vi "onetoteauto.vi"(8 "error in (no error)":errorcluster) -> (0 "error out":errorcluster)   [LabVIEW 2014]
uses:
  <vilib>/Rock Robotics/WPI/Solenoid/WPI_SolenoidValue.ctl
  <vilib>/Rock Robotics/WPI/RobotDrive/WPI_RobotDriveGetSetRefNum.vi
  <vilib>/Rock Robotics/WPI/RobotDrive/WPI_RobotDriveMecanumDrive_Cartesian.vi
  <vilib>/Rock Robotics/WPI/Solenoid/WPI_SolenoidSetEnum.vi
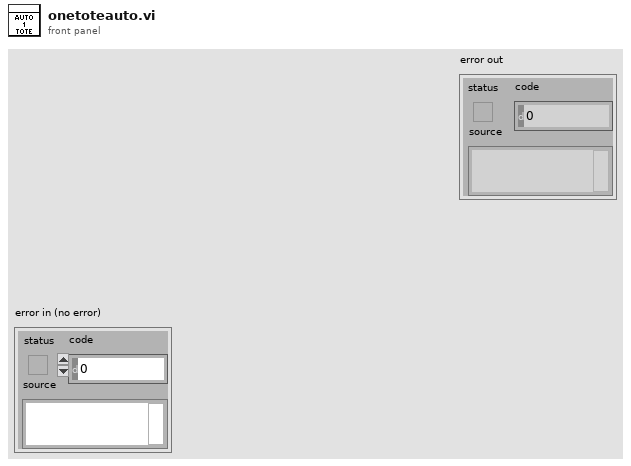
[diagram p1: front panel]
types:
  T1 = typedef "WPI_RobotDriveDevRef.ctl" = cluster{"DevStatus":errorcluster, "Motors[]":T2[], "Square Inputs":bool, "Max Output":dbl}
  T2 = typedef "WPI_MotorControlDeviceRef.ctl" = cluster{"DeviceStatus":errorcluster, "Type":T3, "PWM":cluster{"Controller":T4, "PWM Channel":T5, "DeadBand":T6}, "CAN":cluster{"Device Number":u8, "Control Mode":T7, "Semaphore":T8, "Max Vout":dbl, "TalonSRX Control Mode":T9}, "Invert":bool, "TransformRef":T10, "InvTransformRef":T10}
  T3 = typedef "WPI_MotorControlType.ctl" = enum16{"PWM", "CAN", "CANTalonSRX"}
  T4 = typedef "FPGA_TypedefDigitalModule.ctl" = enum16{"Controller 1"}
  T5 = typedef "FPGA_DIOPWMChannel.ctl" = enum8{"PWM 0", "PWM 1", "PWM 2", "PWM 3", "PWM 4", "PWM 5", "PWM 6", "PWM 7", "PWM 8", "PWM 9", "PWM MXP 0", "PWM MXP 1", "PWM MXP 2", "PWM MXP 3", "PWM MXP 4", "PWM MXP 5", "PWM MXP 6", "PWM MXP 7", "PWM MXP 8", "PWM MXP 9", "Invalid"}
  T6 = typedef "WPI_PWMDeadband.ctl" = cluster{"Name":string, "maxPositivePwm":i32, "minPositivePwm":i32, "centerPwm":i32, "maxNegativePwm":i32, "minNegativePwm":i32, "angularRange":u16}
  T7 = typedef "WPI_CANJaguar_ControlMode.ctl" = enum8{"Percent VBus", "Current", "Speed", "Position", "Voltage"}
  T8 = typedef "Semaphore RefNum" = refnum<k1>
  T9 = typedef "WPI_CANTalonSRX_APIControlMode.ctl" = enum8{"Percent VBus", "Speed", "Position", "Slave", "Unchanged / Invalid"}
  T10 = typedef "WPI_PWMTransform_ConPane.ctl" = refnum<vi>
  T11 = typedef "WPI_SolenoidDevRef.ctl" = cluster{"DevStatus":errorcluster, "Pneumatics Control Module":u8, "Forward Solenoid Channel":T12, "Reverse Solenoid Channel":T12}
  T12 = typedef "WPI_SolenoidChannel.ctl" = enum8{"Solenoid 0", "Solenoid 1", "Solenoid 2", "Solenoid 3", "Solenoid 4", "Solenoid 5", "Solenoid 6", "Solenoid 7", "Invalid"}
  T13 = typedef "WPI_SolenoidValue.ctl" = enum16{"Off", "On", "Forward", "Reverse"}
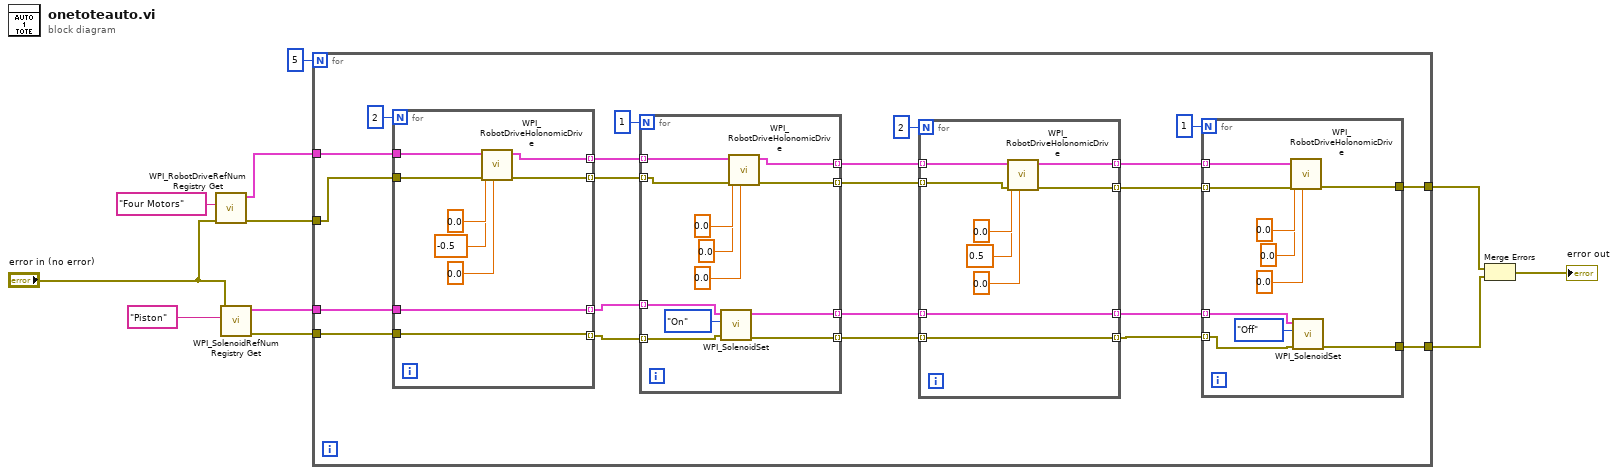
[diagram p0: block diagram]
diagram:
  n1 = call <vilib>:"WPI_RobotDriveRefNum Registry Get.vi"("error in (no error)"="error in (no error)", "refnum name"="Four Motors") -> ("error out"=w8:errorcluster, "RobotDriveDevRef"=w9:T1)  [unwired: 8 in]
  n2 = call <vilib>:"WPI_SolenoidRefNum Registry Get.vi"("error in (no error)"="error in (no error)", "refnum name"="Piston") -> ("error out"=w4:errorcluster, "SolenoidDevRef"=w5:T11)  [unwired: 8 in]
  n3 = for {
    N: 5 -> [_]
    tunnel: w9 -> [w33]
    tunnel: w8 -> [w28]
    tunnel: w5 -> [w24]
    tunnel: w4 -> [w17]
    tunnel: [w13] -> w3
    tunnel: [w12] -> w2
    n4 = for {
      N: 2 -> [_]
      tunnel: w33 -> [w73]
      tunnel: w28 -> [w69]
      tunnel: [w68] -> w27 mode=indexing
      tunnel: [w67] -> w23 mode=indexing
      tunnel: w24 -> [w67]
      tunnel: [w66] -> w20 mode=indexing
      tunnel: [w65] -> w16 mode=indexing
      tunnel: w17 -> [w65]
      n5 = call-poly <vilib>:"WPI_RobotDriveHolonomicDrive.vi"("Rotation"=0.0, "error in (no error)"=w69, "Y"=-0.5, "X"=0.0, "RobotDriveDevRef"=w73) -> ("error out"=w68:errorcluster, "RobotDriveDevRef"=w66:T1)  [unwired: 4 in, 1 out]
    }
    n6 = for {
      N: 1 -> [_]
      tunnel: w27 -> [w61] mode=indexing
      tunnel: [w60] -> w26 mode=indexing
      tunnel: w23 -> [w58] mode=indexing
      tunnel: [w57] -> w21 mode=indexing
      tunnel: w20 -> [w56] mode=indexing
      tunnel: [w55] -> w19 mode=indexing
      tunnel: w16 -> [w54] mode=indexing
      tunnel: [w53] -> w15 mode=indexing
      n7 = call-poly <vilib>:"WPI_SolenoidSet.vi"("error in (no error)"=w54, "Value"=WPI_SolenoidValue."On", "SolenoidDevRef"=w58) -> ("error out"=w53:errorcluster, "SolenoidDevRef"=w57:T11)  [unwired: 7 in]
      n8 = call-poly <vilib>:"WPI_RobotDriveHolonomicDrive.vi"("Rotation"=0.0, "error in (no error)"=w61, "Y"=0.0, "X"=0.0, "RobotDriveDevRef"=w56) -> ("error out"=w60:errorcluster, "RobotDriveDevRef"=w55:T1)  [unwired: 4 in, 1 out]
    }
    n9 = for {
      N: 2 -> [_]
      tunnel: w26 -> [w49] mode=indexing
      tunnel: [w48] -> w25 mode=indexing
      tunnel: [w47] -> w22 mode=indexing
      tunnel: w21 -> [w47] mode=indexing
      tunnel: w19 -> [w46] mode=indexing
      tunnel: [w45] -> w18 mode=indexing
      tunnel: w15 -> [w44] mode=indexing
      tunnel: [w44] -> w14 mode=indexing
      n10 = call-poly <vilib>:"WPI_RobotDriveHolonomicDrive.vi"("Rotation"=0.0, "error in (no error)"=w49, "Y"=0.5, "X"=0.0, "RobotDriveDevRef"=w46) -> ("error out"=w48:errorcluster, "RobotDriveDevRef"=w45:T1)  [unwired: 4 in, 1 out]
    }
    n11 = for {
      N: 1 -> [_]
      tunnel: w25 -> [w40] mode=indexing
      tunnel: w22 -> [w38] mode=indexing
      tunnel: w18 -> [w37] mode=indexing
      tunnel: w14 -> [w36] mode=indexing
      tunnel: [w35] -> w13
      tunnel: [w34] -> w12
      n12 = call-poly <vilib>:"WPI_RobotDriveHolonomicDrive.vi"("Rotation"=0.0, "error in (no error)"=w40, "Y"=0.0, "X"=0.0, "RobotDriveDevRef"=w37) -> ("error out"=w35:errorcluster)  [unwired: 4 in, 2 out]
      n13 = call-poly <vilib>:"WPI_SolenoidSet.vi"("error in (no error)"=w36, "Value"=WPI_SolenoidValue."Off", "SolenoidDevRef"=w38) -> ("error out"=w34:errorcluster)  [unwired: 7 in, 1 out]
    }
  }
  n14 = Merge Errors(w3, w2) -> (→"error out":errorcluster)
